vi "ArduinoLightSwitch_and_TempMonitor.vi"(8 "error in":errorcluster, 10 "Spotlights":bool, 11 "Coaxial light":bool) -> (0 "error out":errorcluster, 3 "Thermometer [C]":dbl(slide) scale=0.0..100.0)   [LabVIEW 2016]
uses:
  <vilib>/LabVIEW Interface for Arduino/Type Defs/Pin Mode.ctl
  <vilib>/LabVIEW Interface for Arduino/LabVIEW Interface for Arduino.lvlib
panel:
  in  "Tab Control":T1(tab)
  in  "Digital I/O Pin - Spotlights":u8=6
  in  "Digital I/O Pin - Coaxial":u8=5
  in  "VCC [V]":dbl=5.0 format="%#_13g"
  out "Waveform Chart":dbl(graph)
  in  "Units (C)":enum16{"Celsius", "Fahrenheit", "Kelvin"}(ring)
  in  "Thermistor Analogue Pin":u8=1
  in  "Paired Resistance (10K Ohms)":dbl=10000.0 format="%#_13g"
  in  "VISA resource":refnum<visa-resource-name>
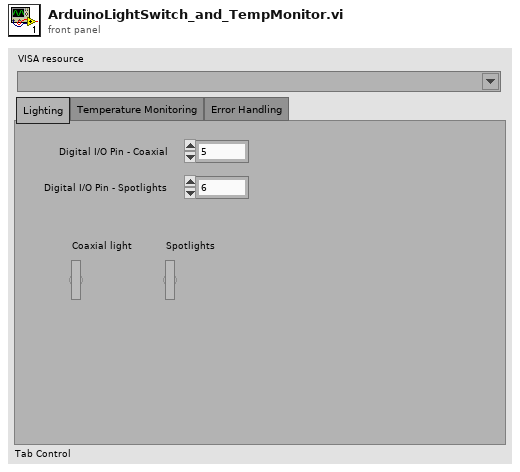
[diagram p1: front panel]
types:
  T1 = enum32{"Lighting", "Temperature Monitoring", "Error Handling"}
  T2 = typedef "LabVIEW Interface for Arduino.lvlib/Pin Mode.ctl" = enum8{"Input", "Output"}
  T3 = typedef "LabVIEW Interface for Arduino.lvlib/Arduino Resource.ctl" = cluster{"VISA resource":refnum<visa-resource-name>, "Board Type":T4, "Connection Type":enum8{"USB / Serial"}, "Bytes Per Packet (15)":u8}
  T4 = typedef "LabVIEW Interface for Arduino.lvlib/Board Type.ctl" = enum16{"Uno", "Dimuelanove w/Atmega 328", "Mega 2560"}
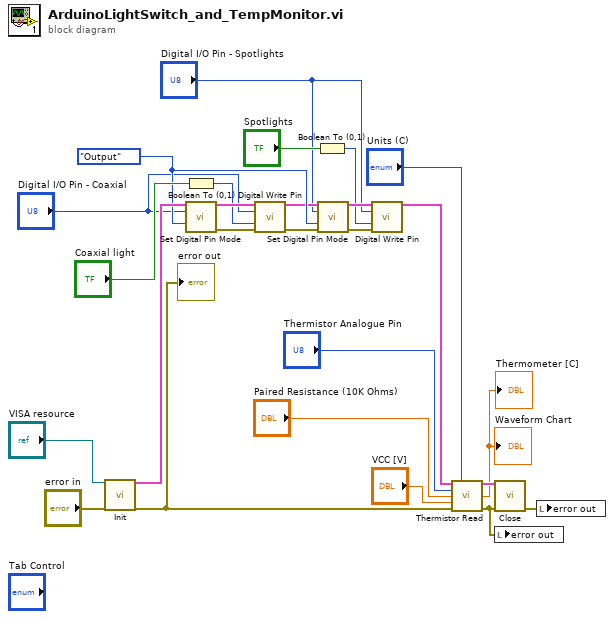
[diagram p0: block diagram]
diagram:
  w10 = Pin_Mode."Output" ("Pin Mode (Input)")
  n1 = call <vilib>:"Init.vi"("VISA resource"="VISA resource", "error in"="error in") -> ("Arduino Resource"=w23:T3, "error out"=w22:errorcluster)  [unwired: 16 in]
  "error out" <- w22
  n2 = Boolean To (0,1)(Boolean="Coaxial light") -> (0, 1=w6:i16)
  n3 = call <vilib>:"Set Digital Pin Mode.vi"("Arduino Resource"=w23, "Digital I/O Pin"="Digital I/O Pin - Coaxial", "Pin Mode (Input)"=w10) -> ("Arduino Resource"=w15:T3, "error out"=w14:errorcluster)  [unwired: 11 in]
  n4 = call <vilib>:"Digital Write Pin.vi"("Arduino Resource"=w15, "Digital I/O Pin (0)"="Digital I/O Pin - Coaxial", "Value (0)"=w6, "error in"=w14) -> ("Arduino Resource"=w9:T3, "error out"=w2:errorcluster)  [unwired: 10 in]
  n5 = Boolean To (0,1)(Boolean="Spotlights") -> (0, 1=w5:i16)
  n6 = call <vilib>:"Set Digital Pin Mode.vi"("Arduino Resource"=w9, "Digital I/O Pin"="Digital I/O Pin - Spotlights", "Pin Mode (Input)"=w10, "error in"=w2) -> ("Arduino Resource"=w13:T3, "error out"=w12:errorcluster)  [unwired: 10 in]
  n7 = call <vilib>:"Digital Write Pin.vi"("Arduino Resource"=w13, "Digital I/O Pin (0)"="Digital I/O Pin - Spotlights", "Value (0)"=w5, "error in"=w12) -> ("Arduino Resource"=w8:T3)  [unwired: 10 in, 1 out]
  n8 = call <vilib>:"Thermistor Read.vi"("Arduino Resource"=w8, "Units (C)"="Units (C)", "Thermistor AI Pin (0)"="Thermistor Analogue Pin", "Paired Resistance (10K Ohms)"="Paired Resistance (10K Ohms)", "Vcc (5 v)"="VCC [V]", "error in"=w22) -> ("Arduino Resource"=w21:T3, "Temperature"=→"Waveform Chart" →"Thermometer [C]":dbl, "error out"=w20:errorcluster)  [unwired: 7 in]
  n9 = call <vilib>:"Close.vi"("Arduino Resource"=w21, "error in"=w20) -> ("error out"=w24:errorcluster)  [unwired: 13 in]
  n10 = local write "error out"(w20) -> ()
  n11 = local write "error out"(w24) -> ()
